vi "ClsRemoveNaN.vi"(2 "Arrayin in":dbl[](array[numeric])) -> (9 "Array Out 2":dbl[](array[numeric]))   [LabVIEW 2015]
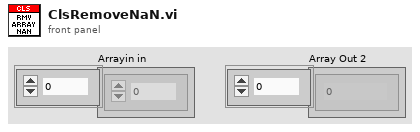
[diagram p1: front panel]
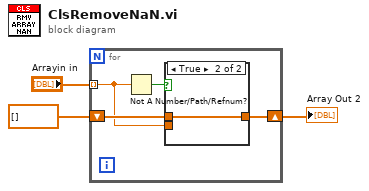
[diagram p0: block diagram]
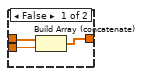
[diagram p2: hidden frame]
diagram:
  n1 = for {
    tunnel: "Arrayin in" -> [w4] mode=indexing
    shift-right: [w5] -> w3
    shift-left: dbl[] [] ("Arrayin 2") -> [w6]
    n2 = Not A Number/Path/Refnum?(number/path/refnum=w4) -> (NaN/Path/Refnum?=w7:bool)
    n3 = case shown="True" w7 {
      tunnel: w6 -> [w10 w11]
      tunnel: [w9 w11] -> w5
      tunnel: w4 -> [w8 _]
      frame False {
        n4 = Build Array (concatenate)(w10, w8) -> (w9:dbl[])
      }
      frame True {
      }
    }
  }
  "Array Out 2" <- w3
